vi "Clear.vi"(8 "error in (no error)":errorcluster, 11 "Mock Log Handler In":refnum<class "Mock Log Handler.lvclass">) -> (0 "error out":errorcluster, 3 "Mock Log Handler Out":refnum<class "Mock Log Handler.lvclass">)   [LabVIEW 2020, in "Mock Log Handler.lvclass"]
doc: "Clears any resorces allocated during initialization."
uses:
  Framework/Base/Base.lvclass/Base.ctl
  Mock Log Handler.lvclass
  Framework/Base/Base.lvclass
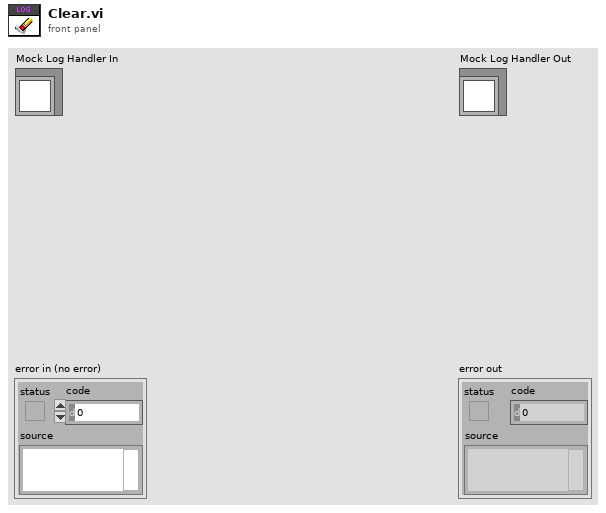
[diagram p1: front panel]
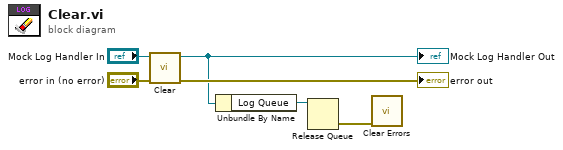
[diagram p0: block diagram]
diagram:
  n1 = call-parent "Clear.vi"("error in (no error)"="error in (no error)", "Base In"="Mock Log Handler In") -> ("error out"=→"error out":errorcluster, "Base Out"=w3:refnum<class "Mock Log Handler.lvclass">)  [unwired: 8 in]
  "Mock Log Handler Out" <- w3
  n2 = Unbundle By Name(w3) -> ("Log Queue"=w2:refnum<queue>)
  n3 = Release Queue(queue=w2) -> (error out=w1:errorcluster)  [unwired: 2 in, 2 out]
  n4 = call <vilib>:"Clear Errors.vi"("error in (no error)"=w1) -> ()  [unwired: 5 in, 2 out]
